vi "figure 2.3.vi"() -> ()   [LabVIEW 2014]
panel:
  out "Numeric":dbl
  in  "OK Button":bool
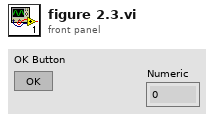
[diagram p1: front panel]
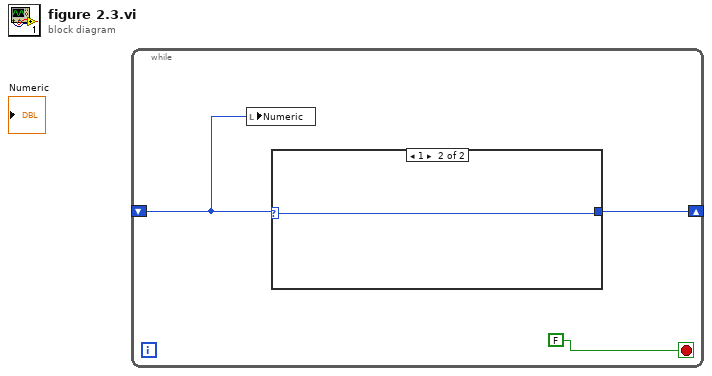
[diagram p0: block diagram]
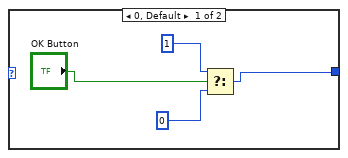
[diagram p2: hidden frame]
diagram:
  n1 = while {
    shift-right: [w3] -> _
    shift-left: _ -> [w2]
    stop <- FALSE stop-if-true
    n2 = local write "Numeric"(w2) -> ()
    n3 = case shown="1" w2 {
      selector: w2 -> [_ w8]
      tunnel: [w5 w8] -> w3
      frame 0, Default {
        n4 = Select(t=1, s="OK Button", f=0) -> (s? t:f=w5:i32)
      }
      frame 1 {
      }
    }
  }
